vi "Import - Buffered Rx Packet.vi"(7 "Rx Packet":T1 {"targetPriority" min=-2 max=16 step=1; "targetProcessor" min=-2 max=16 step=1; "Endianness" items=["big-endian"=0, "little-endian"=2]}, 8 "error in (no error)":errorcluster, 11 "Device Item Ref in":T10 format="%.0x") -> (0 "error out":errorcluster)   [LabVIEW 2016, in "UDP-Custom-Device System Explorer.lvlib"]
uses:
  UDP-Custom-Device System Explorer.lvlib
  <vilib>/NI Veristand/Custom Device API/Custom Device Item Ref.ctl
  Types/XML - New/ImpExp - Rx Packet Data.ctl
  <vilib>/NI Veristand/Custom Device API/Custom Device Item Info.ctl
  Shared/Types/Shared - Channel Data Type.ctl
  Shared/Types/Shared - Buffered.PacketInfo.ctl
  Shared/Types/Shared - Pointer Encoding.ctl
  Shared/Types/Shared - Receive Buffer Options.ctl
  Shared/Types/Shared - Transmit Buffer Options.ctl
  Shared/Types/Shared - New Data Options.ctl
  Types/Threading/Thread Management.ctl
  Property Accessors/Shared Packet Accessors.lvlib
  Property Accessors/Rx Packet Accessors.lvlib
  <vilib>/NI VeriStand/Custom Device API/Custom Device API.lvlib
  Property Accessors/Buffered Data Packet.lvlib
  Shared/UDP-Custom-Device Shared.lvlib
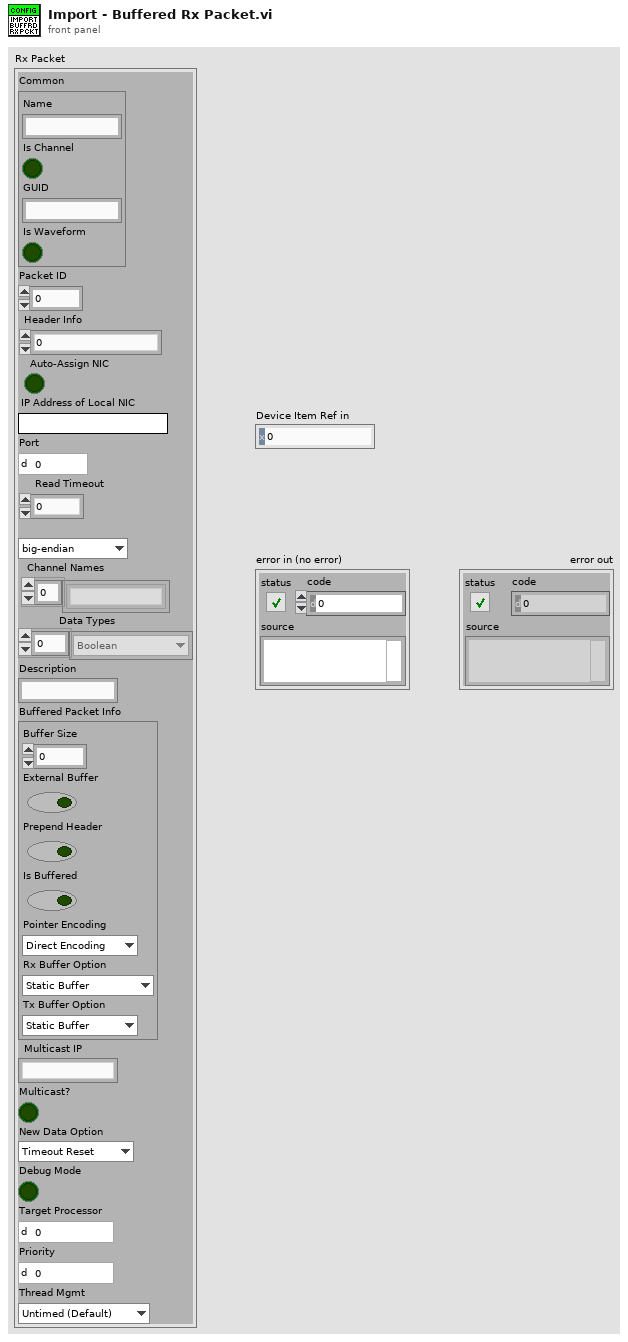
[diagram p1: front panel]
types:
  T1 = typedef "UDP-Custom-Device System Explorer.lvlib/ImpExp - Rx Packet Data.ctl" = cluster{"Common":T2, "Packet ID":i32, "Header Info":u32, "Auto-Assign NIC":bool, "IP Address of Local NIC":string, "Port":u16, "Read Timeout":i32, "Endianness":u16, "Channel Names":string[], "Data Types":T3[], "Description":string, "Buffered Packet Info":T4, "Multicast IP":string, "Multicast?":bool, "New Data Option":T8, "Debug Mode":bool, "targetProcessor":i8, "targetPriority":i16, "Thread Mgmt":T9}
  T2 = typedef "Custom Device API.lvlib/Custom Device Item Info.ctl" = cluster{"Name":string, "Is Channel":bool, "GUID":string, "Is Waveform":bool}
  T3 = typedef "UDP-Custom-Device Shared.lvlib/Shared - Channel Data Type.ctl" = enum16{"Boolean", "Single", "Double", "I8", "I16", "I32", "I64", "U8", "U16", "U32", "U64"}
  T4 = typedef "UDP-Custom-Device Shared.lvlib/Shared - Buffered.PacketInfo.ctl" = cluster{"Buffer Size":i32, "External Buffer":bool, "Prepend Header":bool, "Is Buffered":bool, "Pointer Encoding":T5, "Rx Buffer Option":T6, "Tx Buffer Option":T7}
  T5 = typedef "UDP-Custom-Device Shared.lvlib/Shared - Pointer Encoding.ctl" = enum16{"Direct Encoding", "Conversion Encoding"}
  T6 = typedef "UDP-Custom-Device Shared.lvlib/Shared - Receive Buffer Options.ctl" = enum16{"Static Buffer", "Circular Buffer", "Circular Buffer + Size"}
  T7 = typedef "UDP-Custom-Device Shared.lvlib/Shared - Transmit Buffer Options.ctl" = enum16{"Static Buffer", "FIFO Buffer", "FIFO Buffer + Port"}
  T8 = typedef "UDP-Custom-Device Shared.lvlib/Shared - New Data Options.ctl" = enum16{"Timeout Reset", "Counter"}
  T9 = typedef "UDP-Custom-Device System Explorer.lvlib/Thread Management.ctl" = enum16{"Untimed (Default)", "Timed (High Priority)"}
  T10 = typedef "Custom Device API.lvlib/Custom Device Item Ref.ctl" = u64
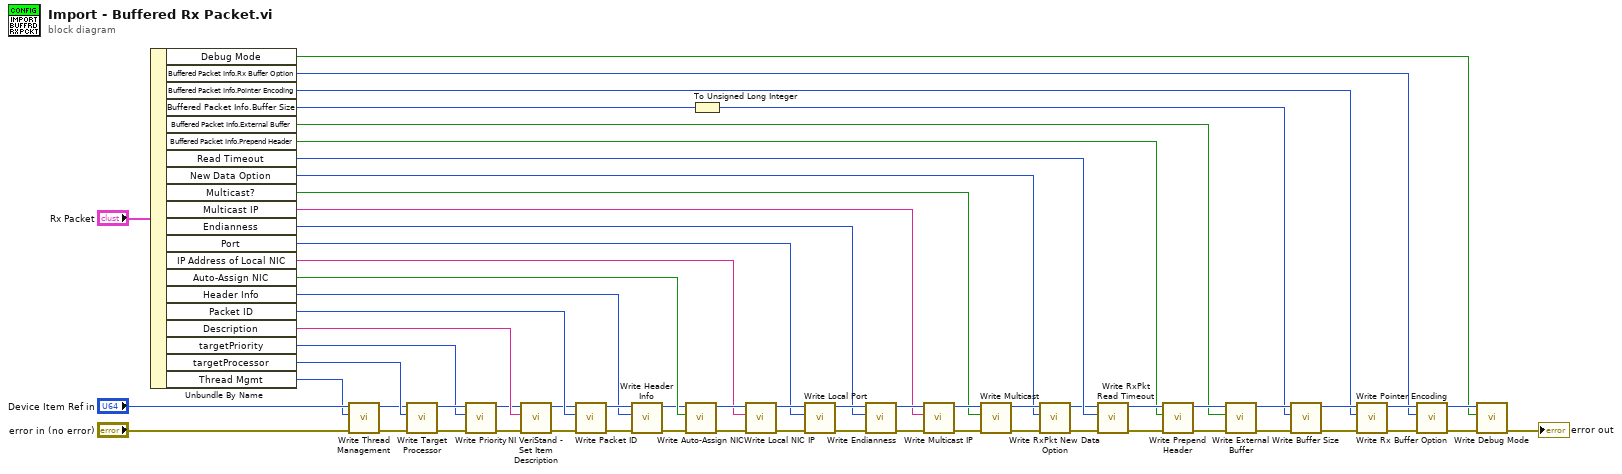
[diagram p0: block diagram]
diagram:
  n1 = Unbundle By Name("Rx Packet") -> ("Debug Mode"=w14:bool, "Buffered Packet Info.Rx Buffer Option"=w16:T6, "Buffered Packet Info.Pointer Encoding"=w24:T5, "Buffered Packet Info.Buffer Size"=w34:i32, "Buffered Packet Info.External Buffer"=w35:bool, "Buffered Packet Info.Prepend Header"=w36:bool, "Read Timeout"=w47:i32, "New Data Option"=w19:T8, "Multicast?"=w27:bool, "Multicast IP"=w28:string, "Endianness"=w48:u16, "Port"=w51:u16, "IP Address of Local NIC"=w54:string, "Auto-Assign NIC"=w58:bool, "Header Info"=w59:u32, "Packet ID"=w62:i32, "Description"=w45:string, "targetPriority"=w9:i16, "targetProcessor"=w8:i8, "Thread Mgmt"=w1:T9)
  n2 = call "Write Thread Management.vi"("error in (no error)"="error in (no error)", "Thread Management"=w1, "Node Ptr"="Device Item Ref in") -> ("error out"=w2:errorcluster, "Node Ptr out"=w4:T10)  [unwired: 7 in]
  n3 = call "Write Target Processor.vi"("error in (no error)"=w2, "targetProcessor"=w8, "Node Ptr"=w4) -> ("error out"=w10:errorcluster, "Node Ptr out"=w11:T10)  [unwired: 7 in]
  n4 = call "Write Priority.vi"("error in (no error)"=w10, "targetPriority"=w9, "Node Ptr"=w11) -> ("error out"=w7:errorcluster, "Node Ptr out"=w6:T10)  [unwired: 7 in]
  n5 = call <vilib>:"NI VeriStand - Set Item Description.vi"("error in (no error)"=w7, "Description"=w45, "Item Ref in"=w6) -> ("error out"=w43:errorcluster, "Item Ref out"=w44:T10)  [unwired: 6 in, 1 out]
  n6 = call "Write Packet ID.vi"("error in (no error)"=w43, "Packet ID"=w62, "Node Ptr"=w44) -> ("error out"=w60:errorcluster, "Node Ptr out"=w61:T10)  [unwired: 7 in]
  n7 = call "Write Header Info.vi"("error in (no error)"=w60, "Header Info"=w59, "Node Ptr"=w61) -> ("error out"=w56:errorcluster, "Node Ptr out"=w57:T10)  [unwired: 7 in]
  n8 = call "Write Auto-Assign NIC.vi"("error in (no error)"=w56, "Auto-Assign NIC"=w58, "Node Ptr"=w57) -> ("error out"=w53:errorcluster, "Node Ptr out"=w55:T10)  [unwired: 7 in]
  n9 = To Unsigned Long Integer(number=w34) -> (unsigned 32bit integer=w33:u32)
  n10 = call "Write Local NIC IP.vi"("error in (no error)"=w53, "IP Address of Local NIC"=w54, "Node Ptr"=w55) -> ("error out"=w50:errorcluster, "Node Ptr out"=w52:T10)  [unwired: 7 in]
  n11 = call "Write Local Port.vi"("error in (no error)"=w50, "Port"=w51, "Node Ptr"=w52) -> ("error out"=w46:errorcluster, "Node Ptr out"=w49:T10)  [unwired: 7 in]
  n12 = call "Write Endianness.vi"("error in (no error)"=w46, "Endianness"=w48, "Node Ptr"=w49) -> ("error out"=w29:errorcluster, "Node Ptr out"=w30:T10)  [unwired: 7 in]
  n13 = call "Write Multicast IP.vi"("error in (no error)"=w29, "Multicast IP Address"=w28, "Node Ptr"=w30) -> ("error out"=w32:errorcluster, "Node Ptr out"=w31:T10)  [unwired: 7 in]
  n14 = call "Write Multicast.vi"("error in (no error)"=w32, "Multicast"=w27, "Node Ptr"=w31) -> ("error out"=w21:errorcluster, "Node Ptr out"=w23:T10)  [unwired: 7 in]
  n15 = call "Write RxPkt New Data Option.vi"("error in (no error)"=w21, "New Data Option"=w19, "Node Ptr"=w23) -> ("error out"=w20:errorcluster, "Node Ptr out"=w22:T10)  [unwired: 7 in]
  n16 = call "Write RxPkt Read Timeout.vi"("error in (no error)"=w20, "Read Timeout"=w47, "Node Ptr"=w22) -> ("error out"=w39:errorcluster, "Node Ptr out"=w42:T10)  [unwired: 7 in]
  n17 = call "Write Prepend Header.vi"("error in (no error)"=w39, "Prepend Header"=w36, "Node Ptr"=w42) -> ("error out"=w38:errorcluster, "Node Ptr out"=w41:T10)  [unwired: 7 in]
  n18 = call "Write External Buffer.vi"("error in (no error)"=w38, "External Buffer"=w35, "Node Ptr"=w41) -> ("error out"=w37:errorcluster, "Node Ptr out"=w40:T10)  [unwired: 7 in]
  n19 = call "Write Buffer Size.vi"("error in (no error)"=w37, "Buffer Size"=w33, "Node Ptr"=w40) -> ("error out"=w26:errorcluster, "Node Ptr out"=w25:T10)  [unwired: 7 in]
  n20 = call "Write Pointer Encoding.vi"("error in (no error)"=w26, "Pointer Encoding"=w24, "Node Ptr"=w25) -> ("error out"=w18:errorcluster, "Node Ptr out"=w17:T10)  [unwired: 7 in]
  n21 = call "Write Rx Buffer Option.vi"("error in (no error)"=w18, "Buffer Option"=w16, "Node Ptr"=w17) -> ("error out"=w13:errorcluster, "Node Ptr out"=w15:T10)  [unwired: 7 in]
  n22 = call "Write Debug Mode.vi"("error in (no error)"=w13, "Debug Mode"=w14, "Node Ptr"=w15) -> ("error out"=→"error out":errorcluster)  [unwired: 7 in, 1 out]
